vi "PH_Countdown-Counter.set i attribute.vi"(0 "i ref in":refnum<vi>, 2 "i attribute":T1={"Machine Time"=[], "Last Shot"=[], "Time since last Shot?"=FALSE, "Calculation"={"Time between Shots [s]"=5400.0, "Ref Remaining Time"=refnum, "Service ID"=-1, "over?"=FALSE, "Ref Time between Shots"=refnum, "Ref Set Mode"=refnum}, "Sound?"=FALSE, "Reminder"={"# 1"={"Pretime [s]"=0.0, "Aktive?"=FALSE, "Over?"=FALSE}, "# 2"={"Pretime [s]"=0.0, "Aktive?"=FALSE, "Over?"=FALSE}}, "MainAmp only"={"State"=TRUE, "GUI Ref"=refnum}}, 5 "error in (no error)":errorcluster) -> (14 "i ref out":refnum<vi>, 19 "error out":errorcluster)   [LabVIEW 2014, in "PH_Countdown-Counter.lvlib"]
doc: "Sets the i attribute data of an object.\n\nLicense Agreement for this software:\n\nCopyright (C)\nGesellschaft für Schwerionenforschung, GSI\nPlanckstr. 1\n64291 Darmstadt\nGermany\n\nContact: D.Beck@gsi.de \n\nThis program is free software; you can redistribute it and/or modify it under the terms of the GNU General Public License as published by the Free Software Foundation; either version 2 of the license, or (at your option) any later version.\n\nThis program is distributed in the hope that it will be useful, but WITHOUT ANY WARRANTY; without even the implied warranty of MERCHANTABILITY or FITNESS FOR A PARTICULAR PURPOSE. See the GNU General License for more details (http://www.gnu.org).\n\nGesellschaft für Schwerionenforschung, GSI\nPlanckstr. 1, 64291 Darmstadt, Germany\nFor all questions and ideas contact: M.Richter@gsi.de, H.Brand@gsi.de or D.Beck@gsi.de.\nLast update: 17-JUN-2004"
uses:
  PH_Countdown-Counter.lvlib
  PH_Countdown-Counter.i attribute.ctl
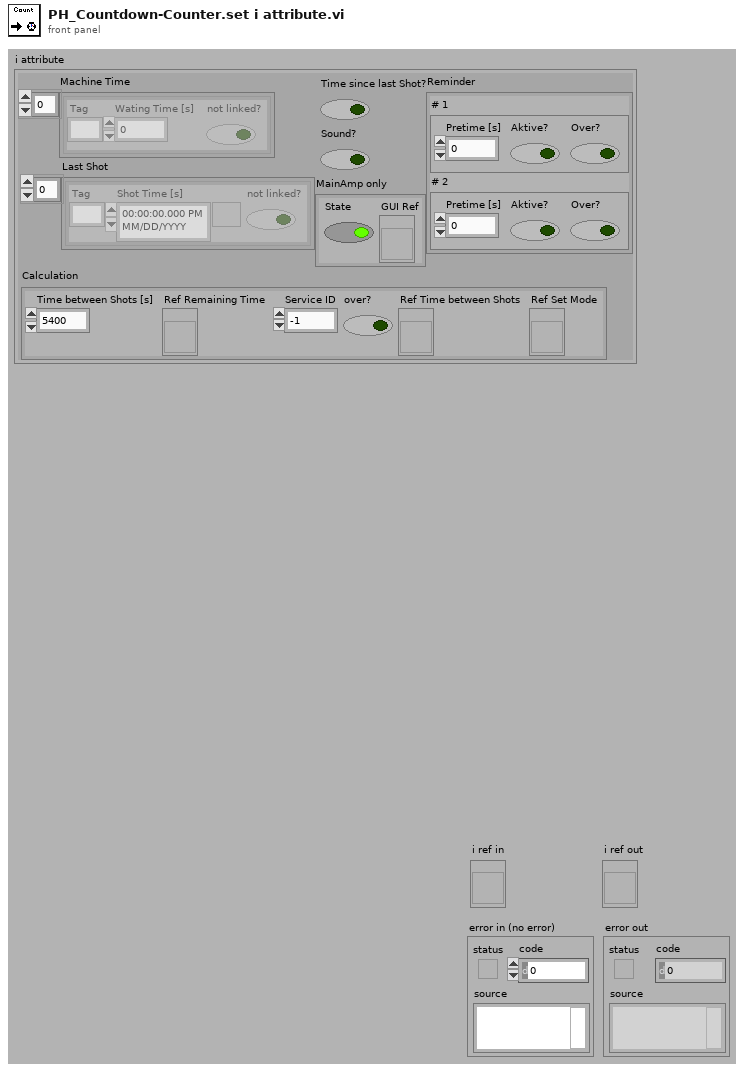
[diagram p1: front panel]
types:
  T1 = typedef "PH_Countdown-Counter.lvlib/PH_Countdown-Counter.i attribute.ctl" = cluster{"Machine Time":cluster{"Tag":string, "Wating Time [s]":dbl, "not linked?":bool}[], "Last Shot":cluster{"Tag":string, "Shot Time [s]":timestamp, "not linked?":bool}[], "Time since last Shot?":bool, "Calculation":cluster{"Time between Shots [s]":dbl, "Ref Remaining Time":refnum<vi>, "Service ID":i32, "over?":bool, "Ref Time between Shots":refnum<vi>, "Ref Set Mode":refnum<vi>}, "Sound?":bool, "Reminder":cluster{"# 1":cluster{"Pretime [s]":dbl, "Aktive?":bool, "Over?":bool}, "# 2":cluster{"Pretime [s]":dbl, "Aktive?":bool, "Over?":bool}}, "MainAmp only":cluster{"State":bool, "GUI Ref":refnum<vi>}}
  T2 = enum16{"SetAttribute", "GetAttribute", "CreateAttribute", "DestroyAttribute", "DestroyAllAtributes"}
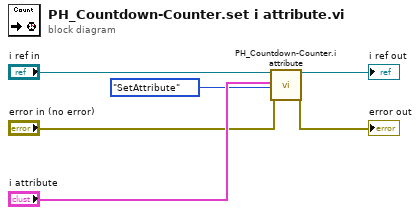
[diagram p0: block diagram]
diagram:
  n1 = call "PH_Countdown-Counter.i attribute.vi"("VI Refnum"="i ref in", "CLASS.i attribute"="i attribute", "Action"=T2."SetAttribute", "error in (no error)"="error in (no error)") -> ("VI Refnum out"=→"i ref out":refnum<vi>, "error out"=→"error out":errorcluster)  [unwired: 13 in, 1 out]
